vi "Register Events.vi"(8 "error in (no error)":errorcluster, 11 "Editor Handler in":refnum<class "Image Editor Handler.lvclass">) -> (0 "error out":errorcluster, 3 "Editor Handler out":refnum<class "Image Editor Handler.lvclass">)   [LabVIEW 2015, in "LV Image Editor Framework.lvlib" / "Image Editor Handler.lvclass"]
uses:
  Image Editor Handler.lvclass
  Forms/Shape/Shape.lvclass
  Image Editor Handler.lvclass/Image Editor Handler.ctl
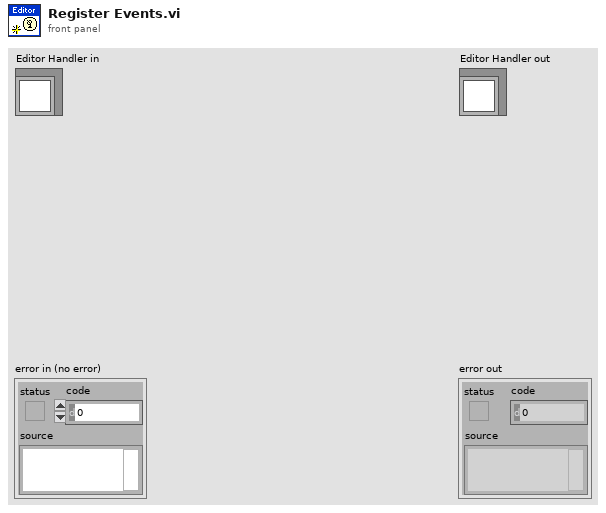
[diagram p1: front panel]
types:
  T1 = cluster{"Shape Reference":refnum<data-value>, "Behind":bool}
  T2 = cluster{"AddShape Data":refnum<user-event>, "Refresh":refnum<user-event>, "Indexes":refnum<user-event>, "Shape Reference":refnum<user-event>, "Shape Reference":refnum<user-event>, "Shape Reference":refnum<user-event>}
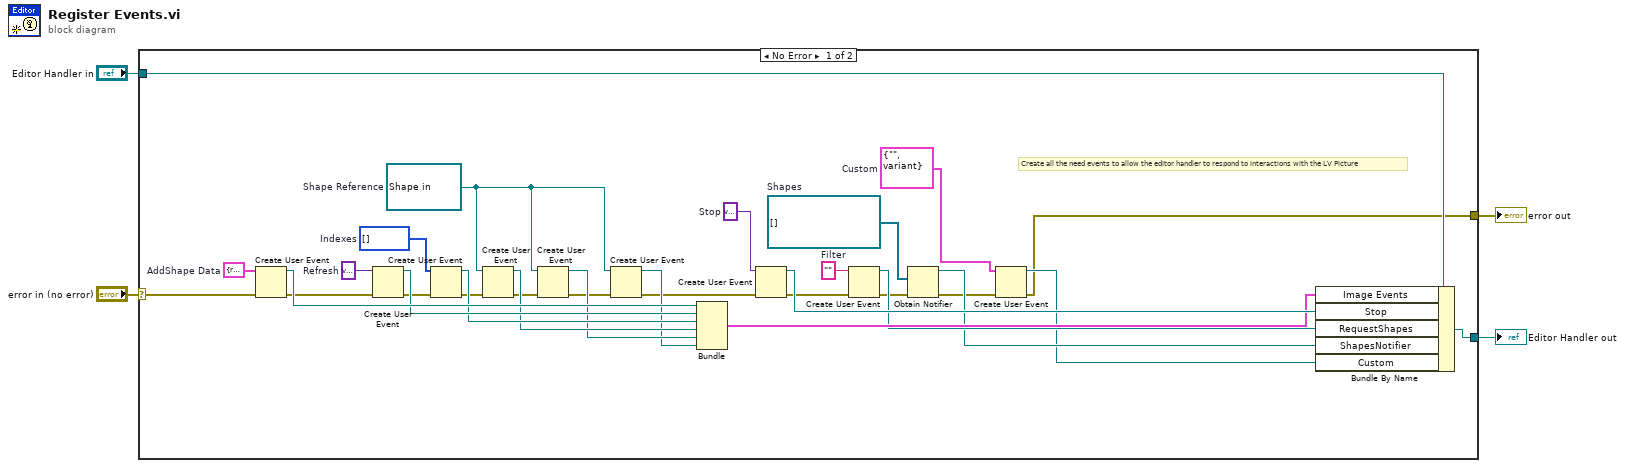
[diagram p0: block diagram]
diagram:
  n1 = case shown="No Error" "error in (no error)" {
    selector: "error in (no error)" -> [w9 w38]
    tunnel: [w10 w38] -> w3
    tunnel: [w33 w37] -> w1
    tunnel: "Editor Handler in" -> [w27 w37]
    frame No Error {
      w13 = cluster{"Cmd":string, "Data":variant} {"Cmd"="", "Data"=variant}  # Custom
      w19 = ""  # Filter
      w17 = refnum<data-value>[] []  # Shapes
      w5 = refnum<data-value> refnum  # Shape Reference
      w26 = i32[] []  # Indexes
      w34 = T1 {"Shape Reference"=refnum, "Behind"=FALSE}  # AddShape Data
      w35 = variant  # Refresh
      w36 = variant  # Stop
      # "Create all the need events to allow the editor handler to respond to interactions with the LV Picture"
      n2 = Create User Event(user event datatype=w34, error in=w9) -> (user event=w31:refnum<user-event>, error out=w28:errorcluster)
      n3 = Create User Event(user event datatype=w35, error in=w28) -> (user event=w30:refnum<user-event>, error out=w25:errorcluster)
      n4 = Create User Event(user event datatype=w26, error in=w25) -> (user event=w24:refnum<user-event>, error out=w22:errorcluster)
      n5 = Create User Event(user event datatype=w5, error in=w22) -> (user event=w23:refnum<user-event>, error out=w21:errorcluster)
      n6 = Create User Event(user event datatype=w5, error in=w21) -> (user event=w20:refnum<user-event>, error out=w7:errorcluster)
      n7 = Create User Event(user event datatype=w5, error in=w7) -> (user event=w8:refnum<user-event>, error out=w6:errorcluster)
      n8 = Bundle("AddShape Data"=w31, "Refresh"=w30, "Indexes"=w24, "Shape Reference"=w23, "Shape Reference"=w20, "Shape Reference"=w8) -> (w29:T2)  [unwired: 1 in]
      n9 = Create User Event(user event datatype=w36, error in=w6) -> (user event=w32:refnum<user-event>, error out=w14:errorcluster)
      n10 = Create User Event(user event datatype=w19, error in=w14) -> (user event=w18:refnum<user-event>, error out=w15:errorcluster)
      n11 = Obtain Notifier(notification data type=w17, error in (no error)=w15) -> (notifier out=w16:refnum<notifier>, error out=w11:errorcluster)  [unwired: 2 in, 1 out]
      n12 = Create User Event(user event datatype=w13, error in=w11) -> (user event=w12:refnum<user-event>, error out=w10:errorcluster)
      n13 = Bundle By Name(cluster=w27, "Image Events"=w29, "Stop"=w32, "RequestShapes"=w18, "ShapesNotifier"=w16, "Custom"=w12) -> (w33:refnum<class "Image Editor Handler.lvclass">)
    }
    frame Error {
    }
  }
  "error out" <- w3
  "Editor Handler out" <- w1
